vi "Vision Server Add Vision Update.vi"(1 "Vision Update":T2, 2 "Vision Server":T1) -> (0 "Vision Server":T1)   [LabVIEW 2016]
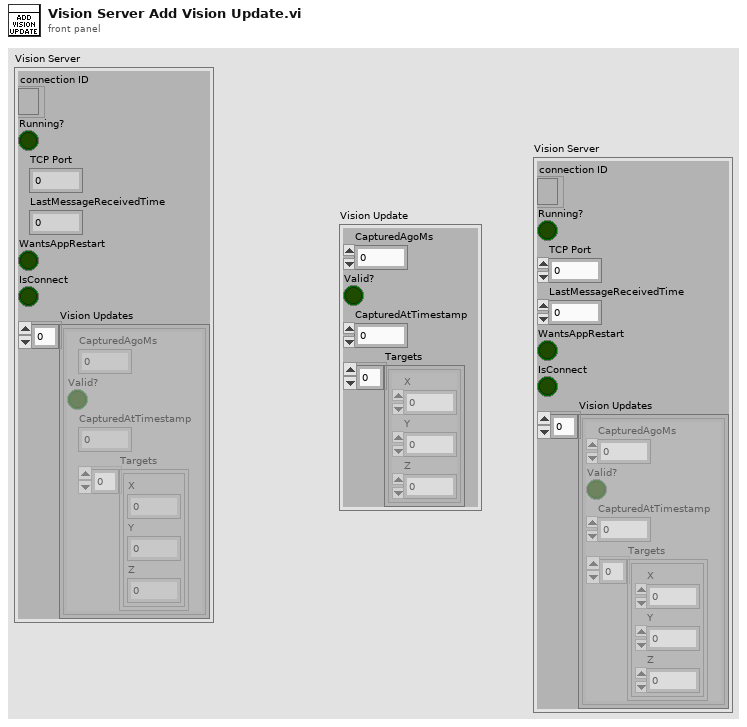
[diagram p1: front panel]
types:
  T1 = cluster{"connection ID":refnum<k5>, "Running?":bool, "TCP Port":u16, "LastMessageReceivedTime":dbl, "WantsAppRestart":bool, "IsConnect":bool, "Vision Updates":cluster{"CapturedAgoMs":i32, "Valid?":bool, "CapturedAtTimestamp":dbl, "Targets":cluster{"X":dbl, "Y":dbl, "Z":dbl}[]}[]}
  T2 = cluster{"CapturedAgoMs":i32, "Valid?":bool, "CapturedAtTimestamp":dbl, "Targets":cluster{"X":dbl, "Y":dbl, "Z":dbl}[]}
  T3 = cluster{"CapturedAgoMs":i32, "Valid?":bool, "CapturedAtTimestamp":dbl, "Targets":cluster{"X":dbl, "Y":dbl, "Z":dbl}[]}[]
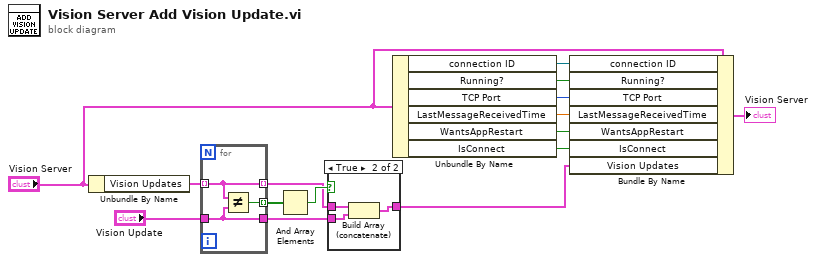
[diagram p0: block diagram]
diagram:
  n1 = Unbundle By Name("Vision Server") -> ("Vision Updates"=w15:T3)
  n2 = for {
    tunnel: w15 -> [w17] mode=indexing
    tunnel: "Vision Update" -> [w16]
    tunnel: [w18] -> w13 mode=indexing
    tunnel: [w17] -> w11 mode=indexing
    tunnel: [w16] -> w10
    n3 = Not Equal?(x=w17, y=w16) -> (x != y?=w18:bool)
  }
  n4 = And Array Elements(Boolean array=w13) -> (logical AND=w12:bool)
  n5 = case shown="True" w12 {
    tunnel: w11 -> [w19 w22]
    tunnel: w10 -> [_ w21]
    tunnel: [w19 w20] -> w3
    frame False {
    }
    frame True {
      n6 = Build Array (concatenate)(w22, w21) -> (w20:T3)
    }
  }
  n7 = Unbundle By Name("Vision Server") -> ("connection ID"=w9:refnum<k5>, "Running?"=w8:bool, "TCP Port"=w7:u16, "LastMessageReceivedTime"=w6:dbl, "WantsAppRestart"=w5:bool, "IsConnect"=w4:bool)
  n8 = Bundle By Name(cluster="Vision Server", "connection ID"=w9, "Running?"=w8, "TCP Port"=w7, "LastMessageReceivedTime"=w6, "WantsAppRestart"=w5, "IsConnect"=w4, "Vision Updates"=w3) -> (→"Vision Server":T1)
